vi "test Merge Import Routing Channels.vi"(8 "error in (no error)":errorcluster, 11 "TestCase in":refnum<class "Routing and Faulting Import Unit Tests.lvclass">) -> (0 "error out":errorcluster, 3 "TestCase out":refnum<class "Routing and Faulting Import Unit Tests.lvclass">)   [LabVIEW 2017, in "Routing and Faulting Import Unit Tests.lvclass"]
uses:
  Routing and Faulting Import Unit Tests.lvclass
  Shared/Channel States.ctl
  Shared/Routing State.ctl
  Shared/Connection.ctl
  Routing and Faulting Import Unit Tests.lvclass/Routing and Faulting Import Unit Tests.ctl
  <userlib>/_OpenG.lib/file/file.llb/Append Path to Root if Relative - Scalar__ogtk.vi
  <vilib>/addons/_JKI Toolkits/VI Tester/TestCase.llb/TestCase.lvclass
  <vilib>/NI/NI VeriStand Custom Device Import and Export Tool/ImportExport.lvlib
  niveristand-custom-device-testing-tools/VeriStandTestUtilities/VeriStandTestUtilities.lvlib
  Scripting/Routing and Faulting Scripting.lvlib
  <vilib>/NI Veristand/Custom Device Tools/Custom Device Utility Library/Custom Device Utility Library.lvlib
  Shared/Routing and Faulting Shared.lvlib
  C:/Program Files (x86)/National Instruments/LabVIEW 2017/vi.lib/addons/_JKI Toolkits/VI Tester/TestCase.llb/TestCase.lvclass
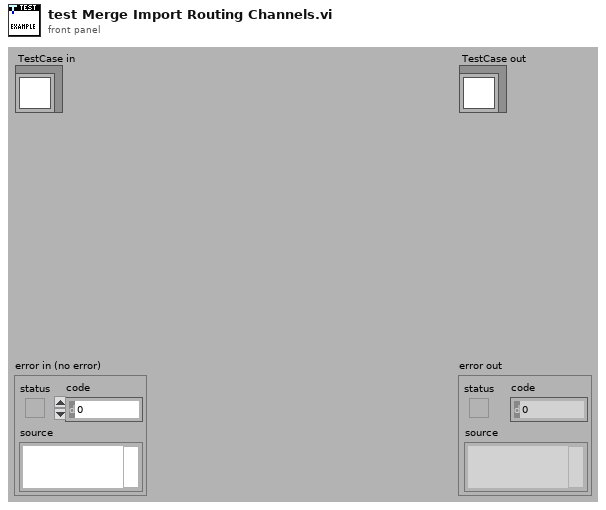
[diagram p1: front panel]
types:
  T1 = typedef "Routing and Faulting Shared.lvlib/Channel States.ctl" = T2[]
  T2 = typedef "Routing and Faulting Shared.lvlib/Routing State.ctl" = cluster{"Name":string, "Description":string, "Value":i32, "Connection List":T3[]}
  T3 = typedef "Routing and Faulting Shared.lvlib/Connection.ctl" = cluster{"Resource":string, "Source":string, "Destination":string}
  T4 = cluster{"Channel Name":string, "Initial State":string, "Description":string, "State Configurations":T1}[]
  T5 = typedef "Custom Device API.lvlib/Custom Device Item Ref.ctl" = u64
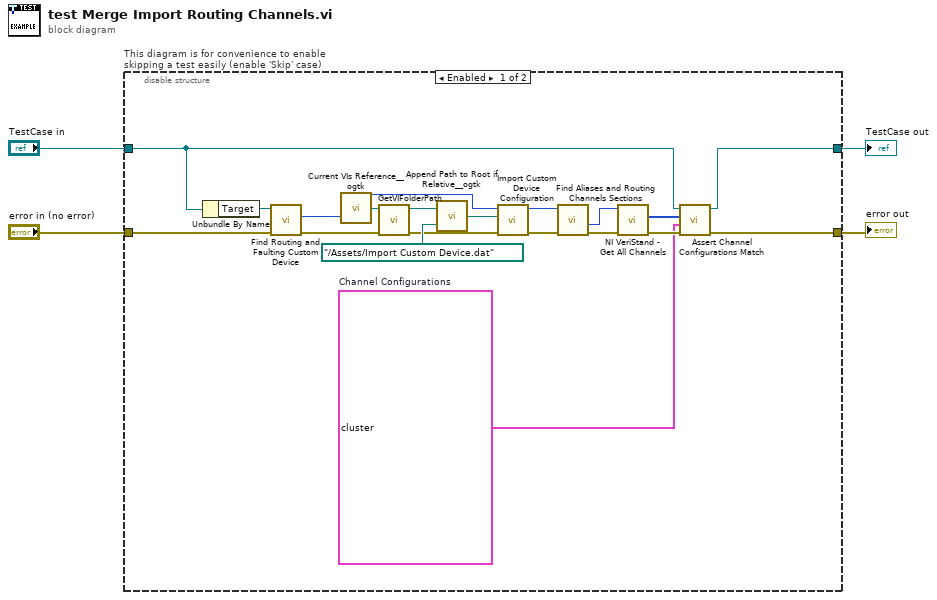
[diagram p0: block diagram]
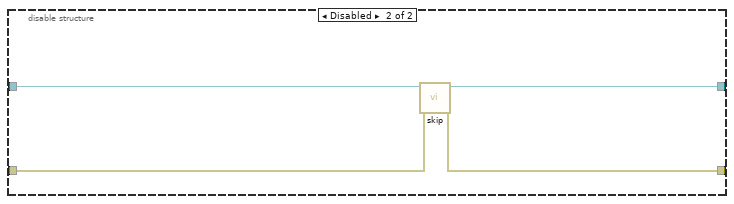
[diagram p2: hidden frame]
diagram:
  n1 = disable-structure "This diagram is for convenience to enable skipping a test easily (enable 'Skip' case)" shown="Enabled" {
    disable-tunnel: "TestCase in" -> [w7 w27]
    disable-tunnel: [w5 w25] -> w1
    disable-tunnel: [w6 w26] -> w3
    disable-tunnel: "error in (no error)" -> [w14 w24]
    frame Enabled {
      w8 = T4 [{"Channel Name"="DefaultValueChan", "Initial State"="", "Description"="Should have default value changed to 0 after import", "State Configurations"=[]}, {"Channel Name"="UnchangedChan", "Initial State"="passThrough", "Description"="Should remain the same after import", "State Configurations"=[{"Name"="passThrough", "Description"="passthrough description", "Value"=23, "Connection List"=[{"Resource"="2010A", "Source"="J1Ch0p", "Destination"="J2Ch16p"}]}, {"Name"="addOne", "Description"="addOne description", "Value"=24, "Connection List"=[{"Resource"="2010A", "Source"="J1Ch0p", "Destination"="J2Ch0p"}, {"Resource"="2010B", "Source"="J1Ch0p", "Destination"="J2Ch0p"}]}]}, {"Channel Name"="StateChangeChan", "Initial State"="passThrough", "Description"="Should have a single state called passThrough after import", "State Configurations"=[{"Name"="passThrough", "Description"="passthrough description", "Value"=23, "Connection List"=[{"Resource"="2010A", "Source"="J1Ch0p", "Destination"="J2Ch16p"}]}]}, {"Channel Name"="ImportedChan", "Initial State"="passThrough", "Description"="Should be added to sysdef after import", "State Configurations"=[{"Name"="passThrough", "Description"="passthrough description", "Value"=23, "Connection List"=[{"Resource"="2010A", "Source"="J1Ch0p", "Destination"="J2Ch16p"}]}, {"Name"="addOne", "Description"="addOne description", "Value"=24, "Connection List"=[{"Resource"="2010A", "Source"="J1Ch0p", "Destination"="J2Ch0p"}, {"Resource"="2010B", "Source"="J1Ch0p", "Destination"="J2Ch0p"}]}]}, {"Channel Name"="StaticChan", "Initial State"="passThrough", "Description"="Should remain the same after import. Does not exist in imported sysdef.", "State Configurations"=[{"Name"="passThrough", "Description"="passthrough description", "Value"=23, "Connection List"=[{"Resource"="2010A", "Source"="J1Ch0p", "Destination"="J2Ch16p"}]}, {"Name"="addOne", "Description"="addOne description", "Value"=24, "Connection List"=[{"Resource"="2010A", "Source"="J1Ch0p", "Destination"="J2Ch0p"}, {"Resource"="2010B", "Source"="J1Ch0p", "Destination"="J2Ch0p"}]}]}]  # Channel Configurations
      n2 = Unbundle By Name(w7) -> ("Target"=w12:refnum<k24>)
      n3 = call "Find Routing and Faulting Custom Device.vi"("error in (no error)"=w14, "Target in"=w12) -> ("error out"=w13:errorcluster, "Routing and Faulting Custom Device Ref"=w11:T5)  [unwired: 7 in, 1 out]
      n4 = call <userlib>:"Current VIs Reference__ogtk.vi"() -> ("Current VI's reference"=w23:refnum<vi>)  [unwired: 5 in]
      n5 = call "GetVIFolderPath.vi"("error in (no error)"=w13, "VI Reference in"=w23) -> ("error out"=w19:errorcluster, "VI Folder Path out"=w22:path)  [unwired: 8 in]
      n6 = call-poly <userlib>:"Append Path to Root if Relative__ogtk.vi"("Absolute or Relative Path"=path "../Assets/Import Custom Device.dat", "Root Path"=w22) -> ("Absolute or Appended Path"=w20:path)
      n7 = call <vilib>:"Import Custom Device Configuration.vi"("error in (no error)"=w19, "Path"=w20, "NodeID"=w11) -> ("error out"=w18:errorcluster, "NodeID out"=w17:u64)  [unwired: 6 in, 1 out]
      n8 = call "Find Aliases and Routing Channels Sections.vi"("error in (no error)"=w18, "Routing and Faulting Custom Device Ref in"=w17) -> ("error out"=w16:errorcluster, "Routing Channels Ref"=w15:T5)  [unwired: 6 in, 2 out]
      n9 = call <vilib>:"NI VeriStand - Get All Channels.vi"("error in"=w16, "Section Ref in"=w15) -> ("error out"=w10:errorcluster, "Channel Refs"=w9:T5[])  [unwired: 6 in, 2 out]
      n10 = call "Assert Channel Configurations Match.vi"("error in (no error)"=w10, "Channel Configurations"=w8, "Channel Refs"=w9, "Test Case in"=w7) -> ("error out"=w6:errorcluster, "Test Case out"=w5:refnum<class "Routing and Faulting Import Unit Tests.lvclass">)  [unwired: 6 in]
    }
    frame Disabled {
      # "skip test result while test is under development"
      n11 = call <vilib>:"skip.vi"("error in (no error)"=w24, "TestCase in"=w27) -> ("error out"=w26:errorcluster, "TestCase out"=w25:refnum<class "Routing and Faulting Import Unit Tests.lvclass">)  [unwired: 8 in]
    }
  }
  "error out" <- w3
  "TestCase out" <- w1
